vi "StopProcess.vi"(0 "reference in":refnum<class "ZeroMQ.lvclass">, 2 "ms timeout (-1)":i32=-1, 5 "error in (no error)":errorcluster) -> (14 "reference out":refnum<class "ZeroMQ.lvclass">, 19 "error out":errorcluster)   [LabVIEW 2018, in "ZeroMQ.lvclass"]
uses:
  ZeroMQ.lvclass
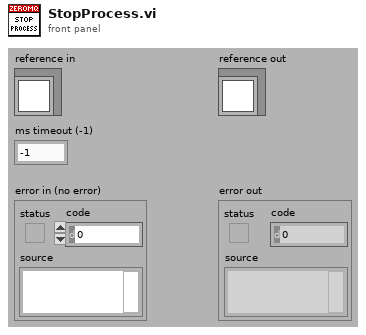
[diagram p1: front panel]
types:
  T1 = enum16{"ReadRepository", "CreateNew", "CreateOrLookUpExisting", "ReadRepositoryAndDestroy"}
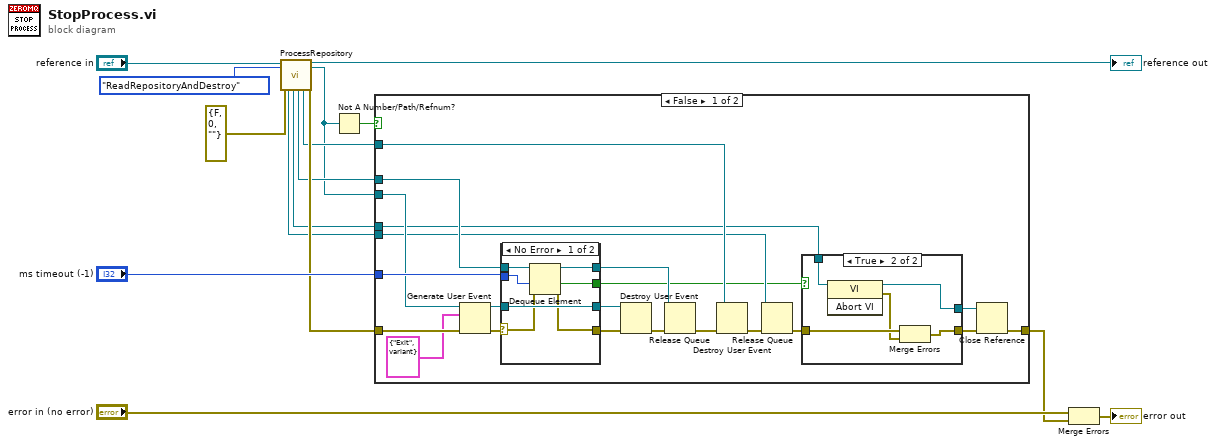
[diagram p0: block diagram]
diagram:
  n1 = call "ProcessRepository.vi"("reference in"="reference in", "Action(ReadRepository)"=T1."ReadRepositoryAndDestroy", "error in (no error)"=errorcluster {"status"=FALSE, "code"=0, "source"=""}) -> ("QueueFromProcess"=w2:refnum<queue>, "ProcessViRef"=w6:refnum<vi>, "ProcessSyncQueue"=w8:refnum<queue>, "EventFromProcess"=w7:refnum<user-event>, "reference out"=→"reference out":refnum<class "ZeroMQ.lvclass">, "EventsToProcess"=w4:refnum<user-event>, "error out"=w9:errorcluster)  [unwired: 9 in, 1 out]
  n2 = Not A Number/Path/Refnum?(number/path/refnum=w4) -> (NaN/Path/Refnum?=w3:bool)
  n3 = case shown="False" w3 {
    tunnel: w8 -> [w36 _]
    tunnel: w9 -> [w28 w54]
    tunnel: [w32 w54] -> w13
    tunnel: w4 -> [w27 _]
    tunnel: "ms timeout (-1)" -> [w31 _]
    tunnel: w7 -> [w29 _]
    tunnel: w6 -> [w25 _]
    tunnel: w2 -> [w21 _]
    frame False {
      n4 = Generate User Event(user event=w27, event data cluster=cluster{"Command":string, "Data":variant} {"Command"="Exit", "Data"=variant} ("event data"), error in=w28) -> (user event out=w35:refnum<user-event>, error out=w30:errorcluster)  [unwired: 1 in]
      n5 = case shown="No Error" w30 {
        tunnel: [w48 w53] -> w34
        tunnel: w36 -> [w47 w51]
        tunnel: [w50 w52] -> w33
        tunnel: w35 -> [w50 w52]
        tunnel: w31 -> [w46 _]
        selector: w30 -> [w49 w53]
        tunnel: [w45 w51] -> w17
        tunnel: [w44 _] -> w16
        frame No Error {
          n6 = Dequeue Element(queue=w47, timeout in ms (-1)=w46, error in (no error)=w49) -> (queue out=w45:refnum<queue>, timed out?=w44:bool, error out=w48:errorcluster)  [unwired: 1 out]
        }
        frame Error {
        }
      }
      n7 = Destroy User Event(user event=w33, error in=w34) -> (error out=w19:errorcluster)
      n8 = Release Queue(queue=w17, error in (no error)=w19) -> (error out=w18:errorcluster)  [unwired: 1 in, 2 out]
      n9 = Destroy User Event(user event=w29, error in=w18) -> (error out=w22:errorcluster)
      n10 = Release Queue(queue=w21, error in (no error)=w22) -> (error out=w20:errorcluster)  [unwired: 1 in, 2 out]
      n11 = case shown="True" w16 {
        tunnel: w25 -> [w37 w43]
        tunnel: [w37 w42] -> w24
        tunnel: [w38 w39] -> w23
        tunnel: w20 -> [w38 w41]
        frame False {
        }
        frame True {
          n12 = invoke class="VI" method="Abort VI"(reference=w43) -> (reference out=w42:refnum<vi>, error out=w40:errorcluster)  [unwired: 2 in, 1 out]
          n13 = Merge Errors(w41, w40) -> (w39:errorcluster)
        }
      }
      n14 = Close Reference(reference=w24, error in (no error)=w23) -> (error out=w32:errorcluster)
    }
    frame True {
    }
  }
  n15 = Merge Errors("error in (no error)", w13) -> (→"error out":errorcluster)
